vi "Read&Write.vi"(6 "In":u8=3 format="%.0x", 9 "Address":u32=262 format="%x", 10 "Read (TRUE)":bool, 11 "address":string="192.168.10.20") -> (0 "error out":errorcluster, 2 "Out":u8=3 format="%.0x")   [LabVIEW 2017]
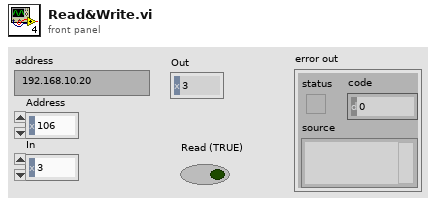
[diagram p1: front panel]
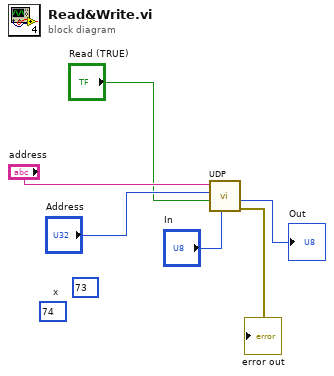
[diagram p0: block diagram]
diagram:
  (unwired) u32 73 ("Address")
  (unwired) u16 74  # x
  n1 = call "UDP.vi"("In"="In", "Read (TRUE)"="Read (TRUE)", "Address"="Address", "IP address"="address") -> ("error out"=→"error out":errorcluster, "Out"=→"Out":u8)  [unwired: 4 in, 1 out]
